vi "Configure Trigger ASK or FSK.vi"(5 "Enable Trigger Delay (F: Disable)":bool, 6 "Trigger Delay Time (0 s)":dbl, 7 "RF Trigger Level (0 dBm)":dbl, 8 "error in (no error)":errorcluster, 9 "Trigger Type (0: Immediate)":i32(ring) items=["Immediate", "External", "RF Trigger"], 10 "External Trigger Type (0: Positive)":i32(ring) items=["Positive", "Negative"], 11 "VISA resource name":refnum<visa-resource-name>) -> (0 "error out":errorcluster, 3 "VISA resource name out":refnum<visa-resource-name>)   [LabVIEW 2022 SP3, in "Agilent N934X Series.lvlib"]
doc: "Configure the trigger settings in ASK and FSK modulation of Demodulation Measurement Type.\n\nNote:\nThis VI is only applicable for N9321C, N9322C, N9323C, N9324C models."
uses:
  <instrlib>/Agilent N934X Series/Agilent N934X Series.lvlib
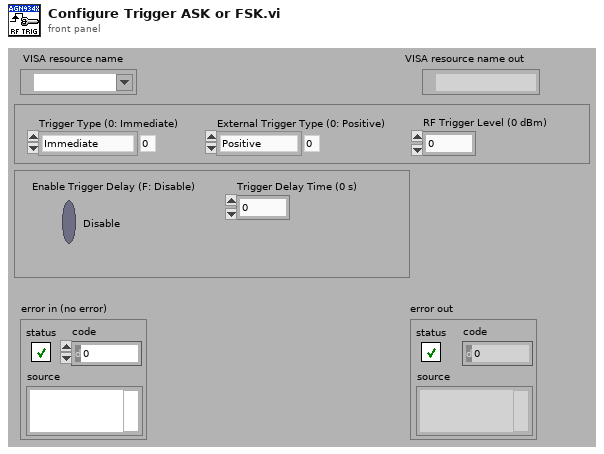
[diagram p1: front panel]
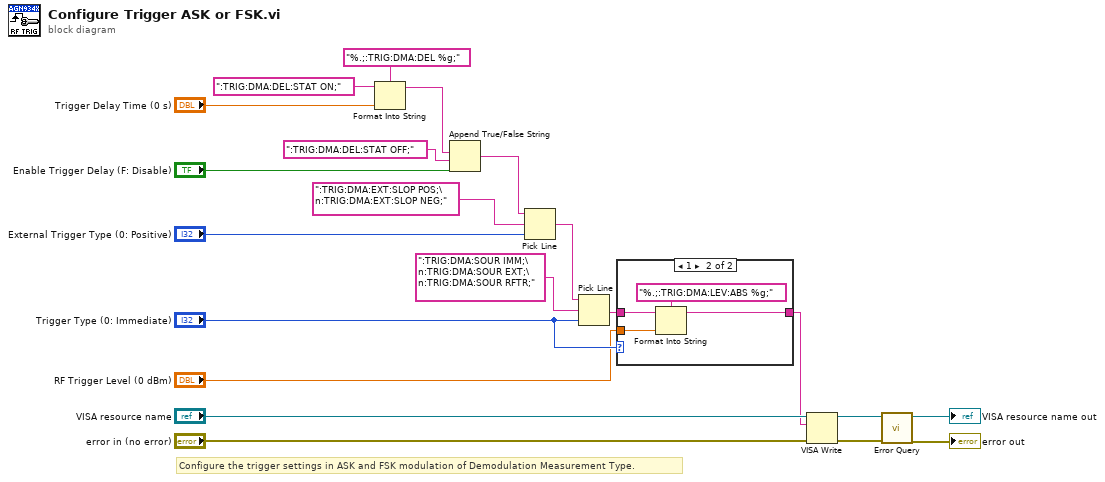
[diagram p0: block diagram]
diagram:
  # "Configure the trigger settings in ASK and FSK modulation of Demodulation Measurement Type."
  n1 = Format Into String(format string="%.;:TRIG:DMA:DEL %g;", initial string=":TRIG:DMA:DEL:STAT ON;", "Trigger Delay Time (0 s)") -> (resulting string=w7:string)  [unwired: 1 in, 1 out]
  n2 = Append True/False String(1:"Enable Trigger Delay (F: Disable)", 2:":TRIG:DMA:DEL:STAT OFF;", 3:w7) -> (0:w15:string)  [unwired: 1 in]
  n3 = Pick Line(string ("")=w15, multi-line string=":TRIG:DMA:EXT:SLOP POS;\n:TRIG:DMA:EXT:SLOP NEG;", line index="External Trigger Type (0: Positive)") -> (output string=w5:string)
  n4 = Pick Line(string ("")=w5, multi-line string=":TRIG:DMA:SOUR IMM;\n:TRIG:DMA:SOUR EXT;\n:TRIG:DMA:SOUR RFTR;", line index="Trigger Type (0: Immediate)") -> (output string=w4:string)
  n5 = case shown="1" "Trigger Type (0: Immediate)" {
    tunnel: w4 -> [w22 w25]
    tunnel: "RF Trigger Level (0 dBm)" -> [_ w24]
    tunnel: [w22 w23] -> w1
    frame 0, 2, Default {
    }
    frame 1 {
      n6 = Format Into String(format string="%.;:TRIG:DMA:LEV:ABS %g;", initial string=w25, w24) -> (resulting string=w23:string)  [unwired: 1 in, 1 out]
    }
  }
  n7 = VISA Write(VISA resource name="VISA resource name", write buffer=w1, error in (no error)="error in (no error)") -> (VISA resource name out=w12:refnum<visa-resource-name>, error out=w11:errorcluster)  [unwired: 1 out]
  n8 = call <instrlib>:"Error Query.vi"("error in (no error)"=w11, "VISA resource name"=w12) -> ("error out"=→"error out":errorcluster, "VISA resource name out"=→"VISA resource name out":refnum<visa-resource-name>)  [unwired: 6 in, 2 out]
